vi "DaqOpen.vi"(9 "scan rate [S/s]":dbl=25000.0 min=0.0 format="%.2f", 11 "physical channels":tag="cDAQ2Mod1/ai0") -> (0 "error out":errorcluster caption="错误输出", 3 "task out":refnum<k21> caption="任务输出")   [LabVIEW 2020]
uses:
  <vilib>/DAQmx/create/channels.llb/DAQmx Create Channel (AI-Voltage-Basic).vi
  <vilib>/DAQmx/configure/timing.llb/DAQmx Timing (Sample Clock).vi
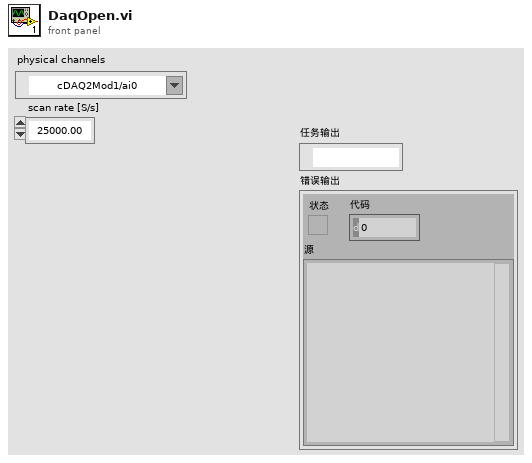
[diagram p1: front panel]
types:
  T1 = cluster{"coupling":i32, "enable excitation":bool, "excitation value":dbl}
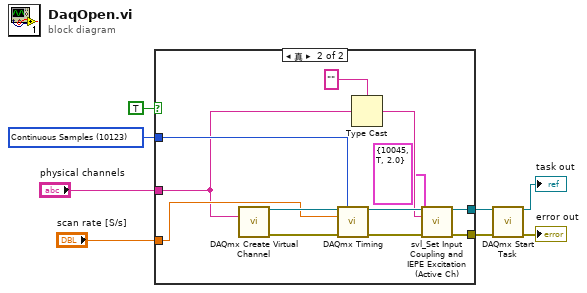
[diagram p0: block diagram]
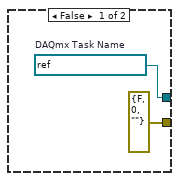
[diagram p2: hidden frame]
diagram:
  w2 = 10123 items=["Finite Samples"=10178, "Continuous Samples"=10123] ("sample mode")
  n1 = case shown="真" TRUE {
    tunnel: [w9 w16] -> w6
    tunnel: [errorcluster {"status"=FALSE, "code"=0, "source"=""} ("error out") w17] -> w5
    tunnel: "scan rate [S/s]" -> [_ w20]
    tunnel: w2 -> [_ w19]
    tunnel: "physical channels" -> [_ w12]
    frame False {
      w9 = refnum<k21> "我的加速度任务"  # DAQmx Task Name
    }
    frame True {
      n2 = call-poly <vilib>:"DAQmx Create Virtual Channel.vi"("physical channels"=w12) -> ("task out"=w22:refnum<k21>, "error out"=w21:errorcluster)  [unwired: 13 in]
      n3 = call-poly <vilib>:"DAQmx Timing.vi"("task/channels in"=w22, "sample mode"=w19, "rate"=w20, "error in"=w21) -> ("task out"=w15:refnum<k21>, "error out"=w18:errorcluster)  [unwired: 10 in]
      n4 = Type Cast(type="", x=w12) -> (*(type *) &x=w13:string)
      n5 = call <vilib>:"svl_Set Input Coupling and IEPE Excitation (Active Ch).vi"("AI task name"=w15, "active channels"=w13, "DSA channel settings"=T1 {"coupling"=10045, "enable excitation"=TRUE, "excitation value"=2.0}, "error in (no error)"=w18) -> ("dup AI task name"=w16:refnum<k21>, "error out"=w17:errorcluster)  [unwired: 10 in]
    }
  }
  n6 = call <vilib>:"DAQmx Start Task.vi"("task/channels in"=w6, "error in"=w5) -> ("task out"=→"task out":refnum<k21>, "error out"=→"error out":errorcluster)  [unwired: 12 in]
